vi "gyro_hand_flag.vi"() -> ()   [LabVIEW 2020]
uses:
  <vilib>/Utility/file.llb/Write Delimited Spreadsheet (string).vi
  <vilib>/Utility/file.llb/Read Delimited Spreadsheet (string).vi
  <vilib>/regexp/Match Regular Expression.xnode
  <vilib>/Analysis/NI_AALBase.lvlib
panel:
  in  "Next":bool
  in  "Tab Control":T1(tab)
  out "csv path":path
  in  "path to ship file":path=path "C:/Users/Lenovo/Desktop/szakdoga"
  in  "path to hand file":path=path "C:/Users/Lenovo/Desktop/szakdoga"
  in  "path to gpx file":path=path "C:/Users/Lenovo/Desktop/szakdoga"
  in  "CSV Filename":string
  out "Offset Graph":cluster{timestamp[], "Y":dbl[]}[](graph)
  out "hand offset out":dbl
  in  "gps offset":dbl
  in  "hand offset":dbl
  in  "x correction thresholds":i32[](array[numeric])=[25, 20, 20, 30]
  out "Threshold Graph":cluster{timestamp[], "Y":dbl[]}[](graph)
  out "x correction thresholds out":i32[](array[numeric])=[25, 20, 20, 30]
  in  "Race time":string
  in  "Other":string
  in  "Orientation":string(combo)
  in  "Ship type":string(combo)
  in  "End Comment":bool
  in  "Type":string(combo)
  out "Timestamp":timestamp
  in  "Flag":string(combo)
  in  "Felvesz":bool
  in  "?":bool
  in  "invert":bool
  out "charge [V]":dbl
  in  "reset":bool
  out "Flag Graph":cluster{timestamp[], "Y":dbl[]}[](graph)
  out "all rows":string[][](array[string])
  # "RESET"
  # "ZOOM"
  # "CURSOR"
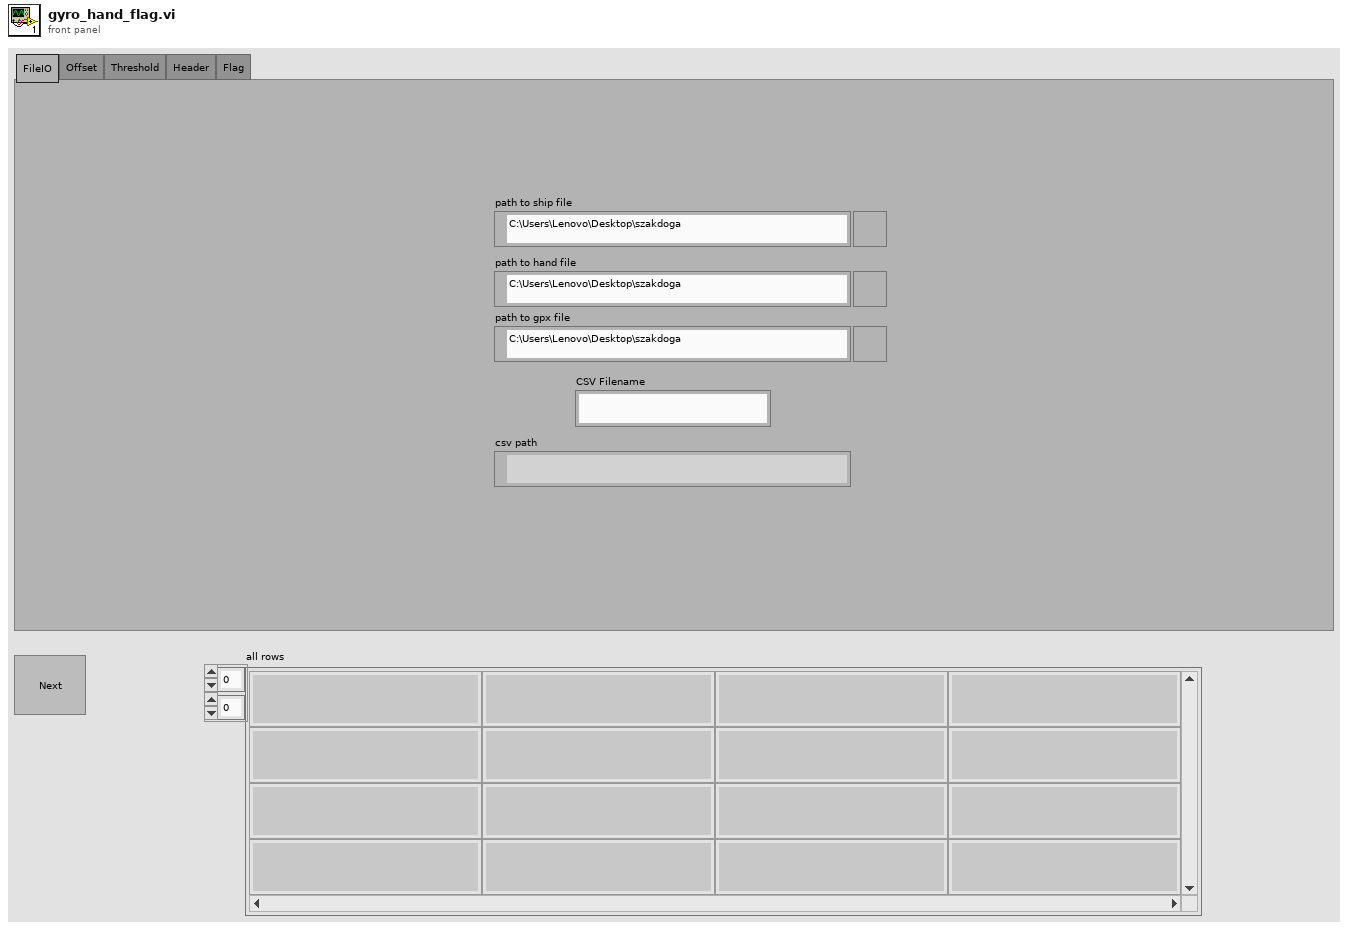
[diagram p1: front panel]
types:
  T1 = enum32{"FileIO", "Offset", "Threshold", "Header", "Flag"}
  T2 = enum16{"open", "replace", "create", "open or create", "replace or create", "replace or create with confirmation"}
  T3 = typedef "gyro_control_measurement_settings.ctl" = cluster{"# Pages":i32, "ODR":u8, "xlRange":u8, "gyroRange":u8, "id":u8, "Samplig Freq [Hz]":dbl, "xlRange in g":dbl, "gyroRange in dps":dbl}
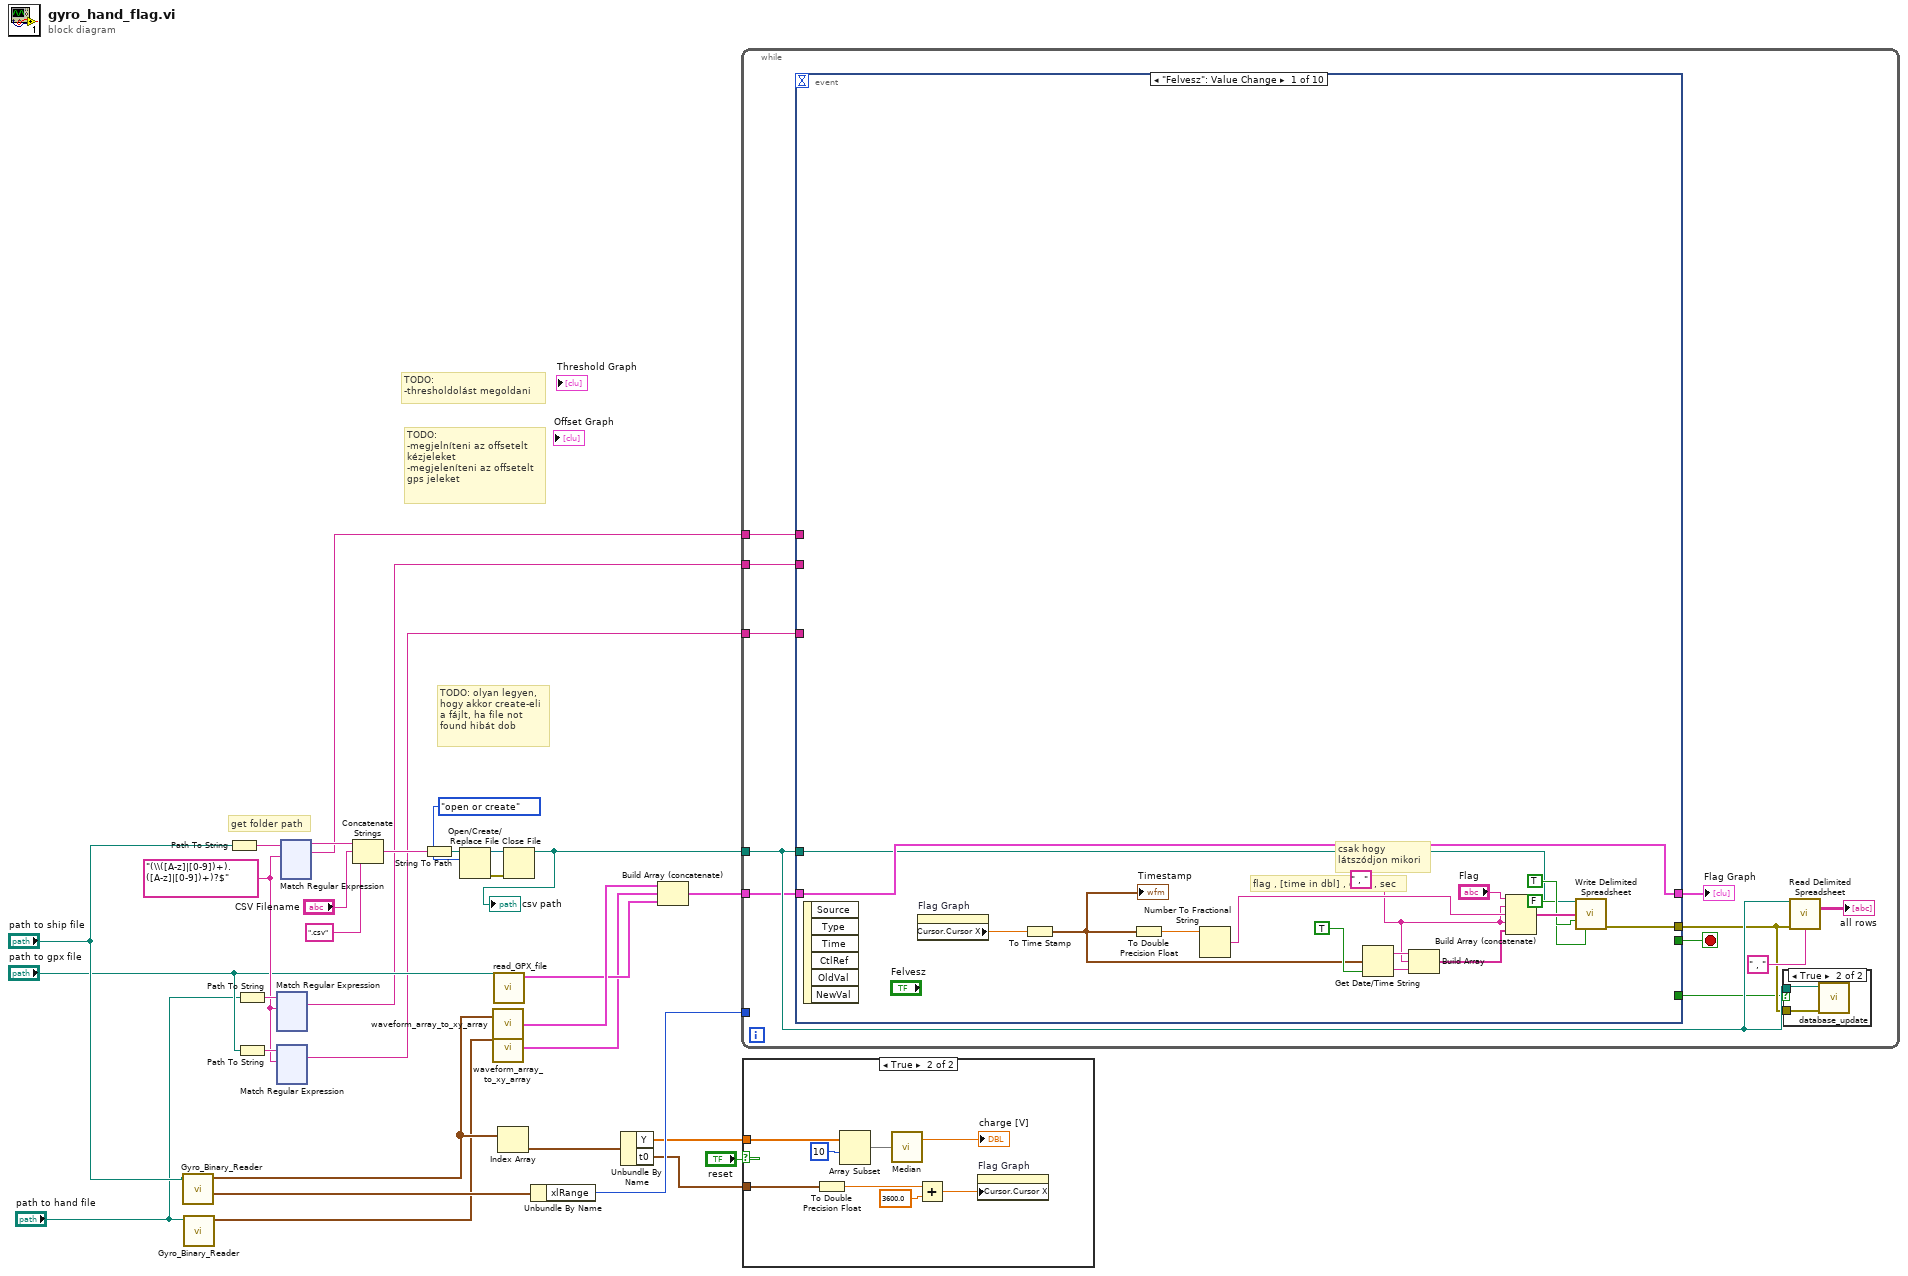
[diagram p0: block diagram]
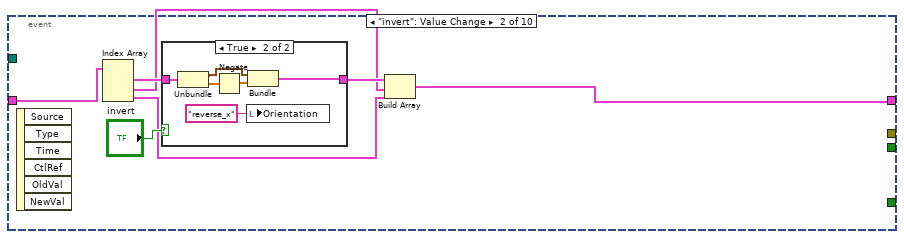
[diagram p4: hidden frame]
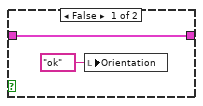
[diagram p5: hidden frame]
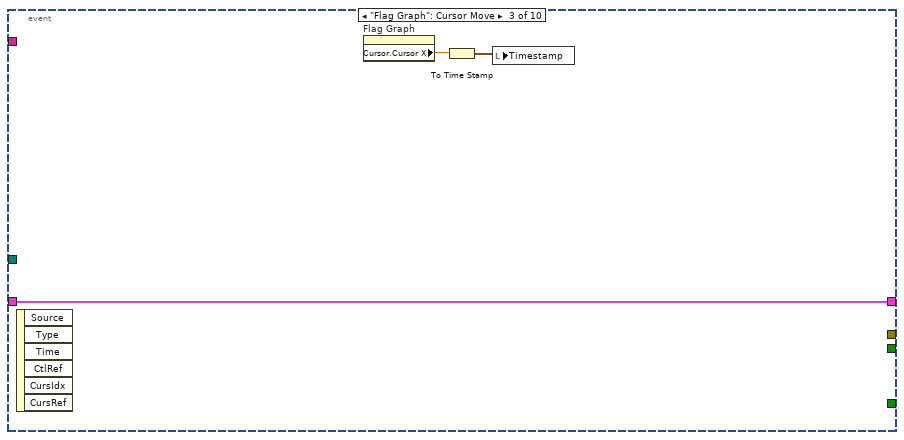
[diagram p6: hidden frame]
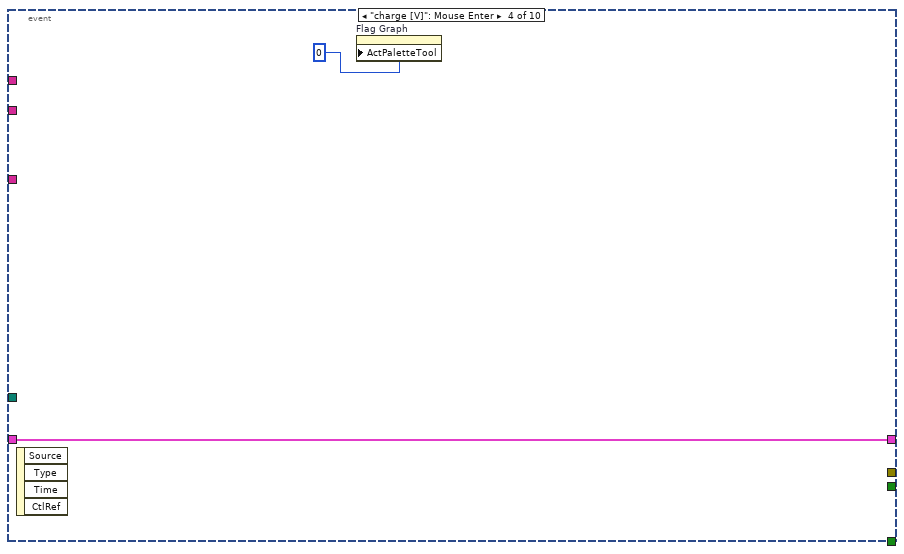
[diagram p7: hidden frame]
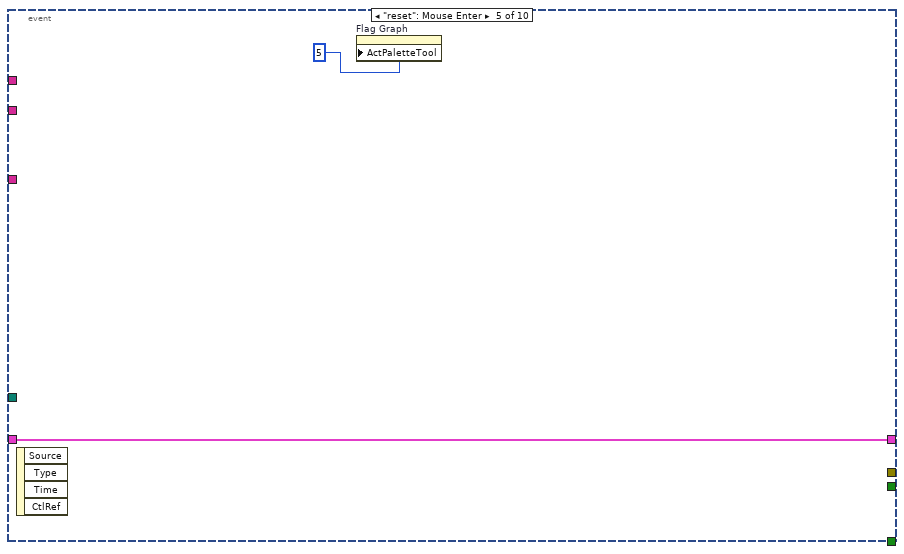
[diagram p8: hidden frame]
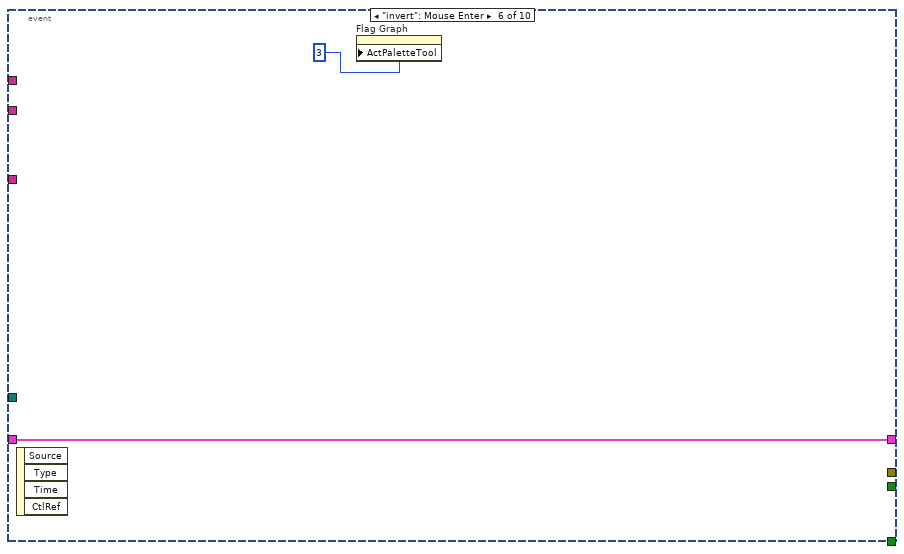
[diagram p9: hidden frame]
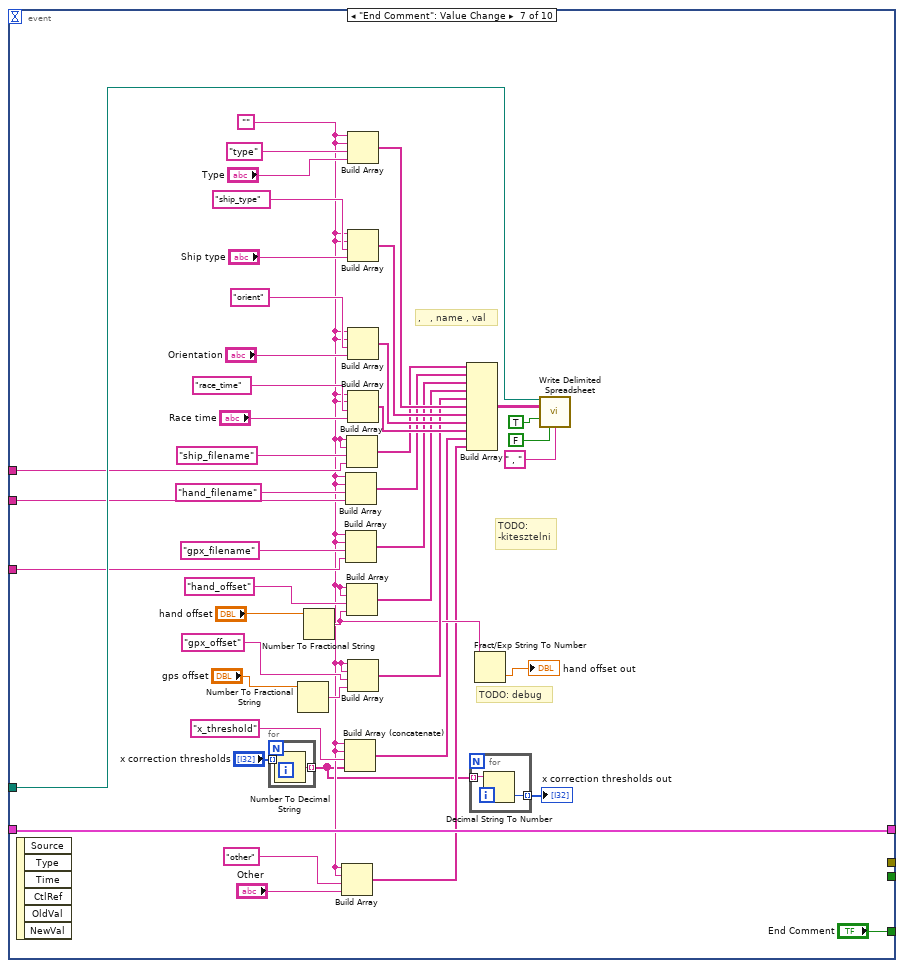
[diagram p10: hidden frame]
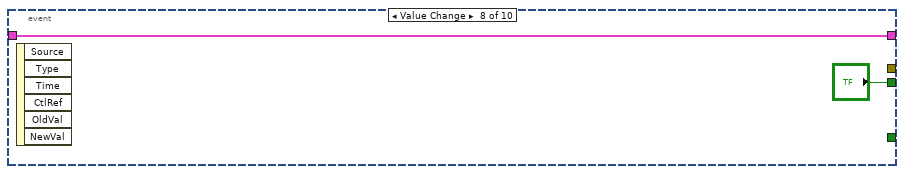
[diagram p11: hidden frame]
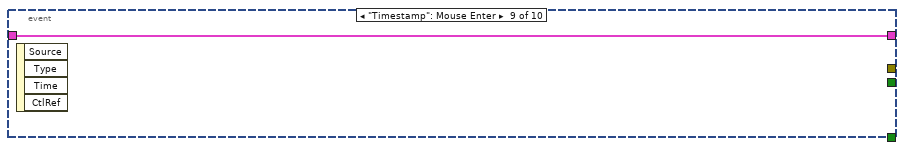
[diagram p12: hidden frame]
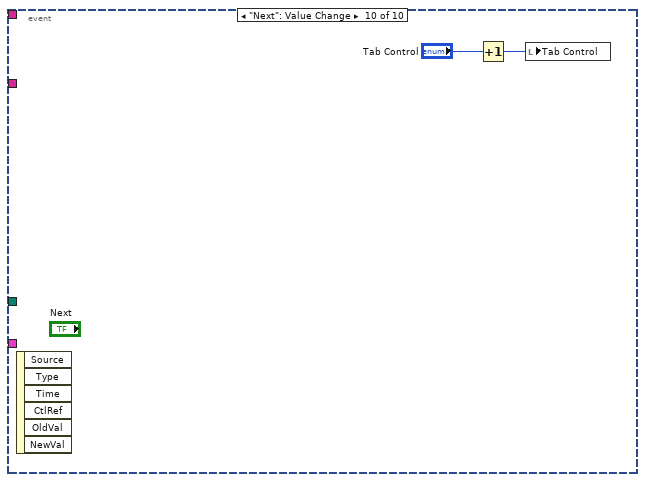
[diagram p13: hidden frame]
diagram:
  w6 = "(\\([A-z]|[0-9])+).([A-z]|[0-9])+)?$" ("regular expression")
  # "TODO:\n-thresholdolást megoldani"
  # "get folder path"
  # "TODO: olyan legyen,  hogy akkor create-eli a fájlt, ha file not found hibát dob"
  # "TODO: \n-megjelníteni az offsetelt\nkézjeleket\n-megjeleníteni az offsetelt\ngps jeleket"
  n1 = call "Gyro_Binary_Reader.vi"("file path (use dialog)"="path to ship file") -> ("Meta"=w22:T3, "Acceleration"=w23:waveform(dbl)[])  [unwired: 7 in, 2 out]
  n2 = call "Gyro_Binary_Reader.vi"("file path (use dialog)"="path to hand file") -> ("Acceleration"=w20:waveform(dbl)[])  [unwired: 7 in, 3 out]
  n3 = Path To String(path="path to ship file") -> (string=w15:string)
  n4 = Path To String(path="path to hand file") -> (string=w8:string)
  n5 = Path To String(path="path to gpx file") -> (string=w7:string)
  n6 = xnode "Match Regular Expression"("input string"=w8, "regular expression"=w6) -> ("whole match"=w3:string)  [unwired: 4 in, 4 out]
  n7 = xnode "Match Regular Expression"("input string"=w7, "regular expression"=w6) -> ("whole match"=w2:string)  [unwired: 4 in, 4 out]
  n8 = xnode "Match Regular Expression"("input string"=w15, "regular expression"=w6) -> ("before match"=w18:string, "whole match"=w1:string)  [unwired: 4 in, 3 out]
  n9 = Concatenate Strings(w18, "CSV Filename", ".csv" ("extension")) -> (w16:string)
  n10 = String To Path(string=w16) -> (path=w13:path)
  n11 = Open/Create/Replace File(file path (use dialog)=w13, operation (0:open)=T2."open or create") -> (refnum out=w10:refnum<file>, error out=w11:errorcluster)  [unwired: 4 in, 1 out]
  n12 = call "waveform_array_to_xy_array.vi"("waveform array"=w23) -> ("XY array"=w25:cluster{timestamp[], "Y":dbl[]}[])  [unwired: 1 in]
  n13 = call "waveform_array_to_xy_array.vi"("waveform array"=w20) -> ("XY array"=w19:cluster{timestamp[], "Y":dbl[]}[])  [unwired: 1 in]
  n14 = call "read_GPX_file.vi"("GPX File Path"="path to gpx file") -> ("XY Speed data"=w24:cluster{timestamp[], dbl[]})  [unwired: 3 in, 3 out]
  n15 = Index Array(array=w23) -> (element=w26:waveform(dbl))  [unwired: 1 in]
  n16 = Close File(refnum=w10, error in=w11) -> (path=w9:path)  [unwired: 1 out]
  "csv path" <- w9
  n17 = Unbundle By Name(w22) -> ("xlRange"=w30:u8)
  n18 = Unbundle By Name(w26) -> ("Y"=w28:dbl[], "t0"=w21:timestamp)
  n19 = Build Array (concatenate)(w25, w19, w24) -> (w29:cluster{timestamp[], "Y":dbl[]}[])
  n20 = while {
    tunnel: w9 -> [w40]
    tunnel: w30 -> [_]
    tunnel: w29 -> [w39]
    tunnel: w3 -> [w34]
    tunnel: w2 -> [w33]
    tunnel: w1 -> [w32]
    stop <- w42 stop-if-true
    n21 = event shown="[0] \"Felvesz\": Value Change" {
      selector: _ -> [_ _ _ _ _ _ _ _ _ _]
      dyn-events: _ -> [_ _ _ _ _ _ _ _ _ _]
      timeout: _ -> [_ _ _ _ _ _ _ _ _ _]
      tunnel: [_ _ _ _ _ _ _ "?" _ _] -> w42
      tunnel: w40 -> [w46 _ _ _ _ _ w128 _ _ _]
      tunnel: [w45 _ _ _ _ _ _ _ _ _] -> w38
      tunnel: w39 -> [w47 w67 w76 w79 w81 w83 w111 w135 w137 _]
      tunnel: [w47 w61 w76 w79 w81 w83 w111 w135 w137 _] -> w35
      tunnel: [_ _ _ _ _ _ "End Comment" _ _ _] -> w37
      tunnel: w34 -> [_ _ _ _ _ _ w108 _ _ _]
      tunnel: w33 -> [_ _ _ _ _ _ w106 _ _ _]
      tunnel: w32 -> [_ _ _ _ _ _ w93 _ _ _]
      event "Felvesz": Value Change {
        w54 = " , " ("element")
        # "csak hogy \nlátszódjon mikori"
        # "flag , [time in dbl] , date , sec"
        n22 = event-data() -> ()  [unwired: 1 in, 6 out]
        n23 = property on="Flag Graph" class="XYGraph (strict)"() -> ("Cursor.Cursor X"=w49:dbl)  [unwired: 2 in, 2 out]
        n24 = To Time Stamp(1:w49) -> (0:w48:timestamp)
        "Timestamp" <- w48
        n25 = To Double Precision Float(number=w48) -> (double precision float=w59:dbl)
        n26 = Number To Fractional String(number=w59) -> (F-format string=w60:string)  [unwired: 3 in]
        n27 = Get Date/Time String(seconds (now)=w48, want seconds? (F)=TRUE) -> (date string=w56:string, time string=w57:string)  [unwired: 1 in]
        n28 = Build Array(w56, w54, w57) -> (w58:string[])
        n29 = Build Array (concatenate)("Flag", w54, w60, w54, w58) -> (w55:string[])
        n30 = call-poly <vilib>:"Write Delimited Spreadsheet.vi"("file path (dialog if empty)"=w46, "1D data"=w55, "append to file? (new file:F)"=TRUE, "transpose? (no:F)"=FALSE) -> ("error out"=w45:errorcluster)  [unwired: 10 in, 1 out]
      }
      event "invert": Value Change {
        n31 = event-data() -> ()  [unwired: 1 in, 6 out]
        n32 = Index Array(array=w67) -> (element #1=w65:cluster{timestamp[], "Y":dbl[]}, element #2=w63:cluster{timestamp[], "Y":dbl[]}, element #3=w62:cluster{timestamp[], "Y":dbl[]})  [unwired: 3 in]
        n33 = case shown="True" "invert" {
          tunnel: w65 -> [w69 w75]
          tunnel: [w69 w73] -> w64
          frame False {
            n34 = local write "Orientation"("ok" ("Orientation")) -> ()
          }
          frame True {
            n35 = Unbundle(w75) -> (w71:timestamp[], "Y"=w74:dbl[])
            n36 = Negate(x=w74) -> (-x=w72:dbl[])
            n37 = local write "Orientation"("reverse_x" ("Orientation")) -> ()
            n38 = Bundle(w71, w72) -> (w73:cluster{timestamp[], dbl[]})  [unwired: 1 in]
          }
        }
        n39 = Build Array(w64, w63, w62) -> (w61:cluster{timestamp[], "Y":dbl[]}[])
      }
      event "Flag Graph": Cursor Move {
        n40 = event-data() -> ()  [unwired: 1 in, 6 out]
        n41 = property on="Flag Graph" class="XYGraph (strict)"() -> ("Cursor.Cursor X"=w77:dbl)  [unwired: 2 in, 2 out]
        n42 = To Time Stamp(1:w77) -> (0:w78:timestamp)
        n43 = local write "Timestamp"(w78) -> ()
      }
      event "charge [V]": Mouse Enter {
        n44 = event-data() -> ()  [unwired: 1 in, 4 out]
        n45 = property on="Flag Graph" class="XYGraph (strict)"("ActPaletteTool"=0 ("Palette:Active Tool")) -> ()  [unwired: 2 in, 2 out]
      }
      event "reset": Mouse Enter {
        n46 = event-data() -> ()  [unwired: 1 in, 4 out]
        n47 = property on="Flag Graph" class="XYGraph (strict)"("ActPaletteTool"=5 ("Palette:Active Tool")) -> ()  [unwired: 2 in, 2 out]
      }
      event "invert": Mouse Enter {
        n48 = event-data() -> ()  [unwired: 1 in, 4 out]
        n49 = property on="Flag Graph" class="XYGraph (strict)"("ActPaletteTool"=3 ("Palette:Active Tool")) -> ()  [unwired: 2 in, 2 out]
      }
      event "End Comment": Value Change {
        w88 = ""
        # "TODO: debug"
        # "TODO:\n-kitesztelni"
        # ",   , name , val"
        n50 = event-data() -> ()  [unwired: 1 in, 6 out]
        n51 = for {
          tunnel: "x correction thresholds" -> [w134] mode=indexing
          tunnel: [w133] -> w86 mode=indexing
          n52 = Number To Decimal String(number=w134) -> (decimal integer string=w133:string)  [unwired: 1 in]
        }
        n53 = Number To Fractional String(number="gps offset") -> (F-format string=w96:string)  [unwired: 3 in]
        n54 = Number To Fractional String(number="hand offset") -> (F-format string=w99:string)  [unwired: 3 in]
        n55 = Build Array(w88, w88, "other", "Other") -> (w87:string[])
        n56 = Build Array (concatenate)(w88, w88, "x_threshold", w86) -> (w90:string[])
        n57 = Build Array(w88, w88, "hand_filename", w108) -> (w105:string[])
        n58 = Build Array(w88, w88, "gpx_filename", w106) -> (w104:string[])
        n59 = Build Array(w88, w88, "ship_filename", w93) -> (w92:string[])
        n60 = Build Array(w88, w88, "hand_offset", w99) -> (w102:string[])
        n61 = Build Array(w88, w88, "type", "Type") -> (w121:string[])
        n62 = Build Array(w88, w88, "ship_type", "Ship type") -> (w120:string[])
        n63 = Build Array(w88, w88, "orient", "Orientation") -> (w116:string[])
        n64 = Build Array(w88, w88, "race_time", "Race time") -> (w115:string[])
        n65 = Build Array(w88, w88, "gpx_offset", w96) -> (w101:string[])
        n66 = Build Array(w92, w105, w104, w102, w101, w121, w120, w116, w115, w90, w87) -> (w126:string[][])
        n67 = for {
          tunnel: w86 -> [w132] mode=indexing
          tunnel: [w131] -> w85 mode=indexing
          n68 = Decimal String To Number(string=w132) -> (number=w131:i32)  [unwired: 2 in, 1 out]
        }
        "x correction thresholds out" <- w85
        n69 = Fract/Exp String To Number(string=w99) -> (number=→"hand offset out":dbl)  [unwired: 3 in, 1 out]
        n70 = call-poly <vilib>:"Write Delimited Spreadsheet.vi"("file path (dialog if empty)"=w128, "2D data"=w126, "append to file? (new file:F)"=TRUE, "transpose? (no:F)"=FALSE, "delimiter (\\t)"=" , " ("element")) -> ()  [unwired: 9 in, 2 out]
      }
      event Value Change {
        n71 = event-data() -> ()  [unwired: 1 in, 6 out]
      }
      event "Timestamp": Mouse Enter {
        n72 = event-data() -> ()  [unwired: 1 in, 4 out]
      }
      event "Next": Value Change {
        n73 = event-data() -> ()  [unwired: 1 in, 6 out]
        n74 = Increment(x="Tab Control") -> (x+1=w138:T1)
        n75 = local write "Tab Control"(w138) -> ()
      }
    }
    "Flag Graph" <- w35
    n76 = case shown="True" w37 {
      tunnel: w40 -> [_ w44]
      tunnel: w38 -> [_ w43]
      frame False {
      }
      frame True {
        n77 = call "database_update.vi"("error in (no error)"=w43, "path to csv file"=w44) -> ()  [unwired: 10 in]
      }
    }
    n78 = call-poly <vilib>:"Read Delimited Spreadsheet.vi"("file path (dialog if empty)"=w40, "error in (no error)"=w38, "delimiter (\\t)"=" , " ("delimiter (\\t)")) -> ("all rows"=→"all rows":string[][])  [unwired: 7 in, 5 out]
  }
  n79 = case shown="True" "reset" {
    tunnel: w21 -> [_ w145]
    tunnel: w28 -> [_ w144]
    frame False {
    }
    frame True {
      n80 = To Double Precision Float(number=w145) -> (double precision float=w146:dbl)
      n81 = Array Subset(array=w144, index=10) -> (w143:dbl[])  [unwired: 1 in]
      n82 = call <vilib>:"Median.vi"("X"=w143) -> ("median"=→"charge [V]":dbl)  [unwired: 1 out]
      n83 = Add(x=w146, y=3600.0) -> (x+y=w140:dbl)
      n84 = property on="Flag Graph" class="XYGraph (strict)"("Cursor.Cursor X"=w140) -> ()  [unwired: 2 in, 2 out]
    }
  }
